vi "Save to binary file.vi"(6 "# saved frames out in":i32, 9 "Saving File":bool, 10 "Image array":u16[](array[numeric]), 11 "Byte Stream File in":refnum<file>) -> (2 "# saved frames out out":i32, 3 "Byte Stream File out":refnum<file>)   [LabVIEW 2011]
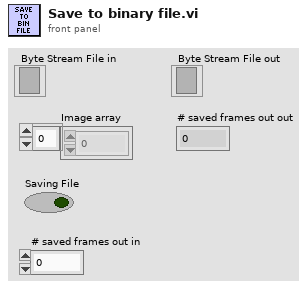
[diagram p1: front panel]
types:
  T1 = enum16{"big-endian, network order", "native, host order", "little-endian"}
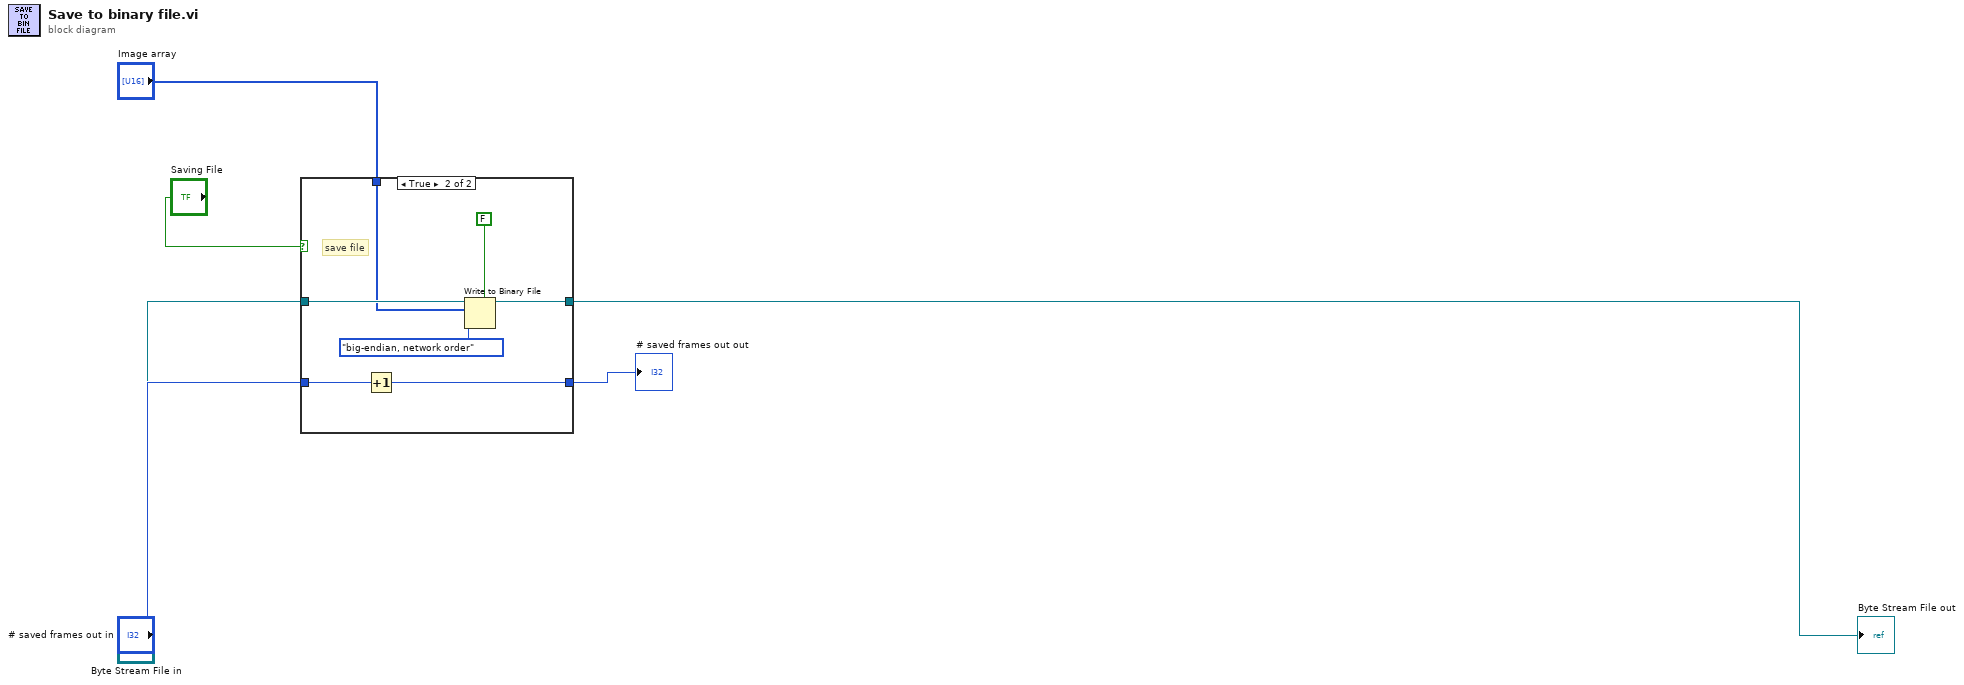
[diagram p0: block diagram]
diagram:
  n1 = case shown="True" "Saving File" {
    tunnel: [w8 w15] -> w1
    tunnel: "Byte Stream File in" -> [w8 w14]
    tunnel: "Image array" -> [_ w13]
    tunnel: "# saved frames out in" -> [w7 w10]
    tunnel: [w7 w9] -> w5
    frame False {
    }
    frame True {
      # "save file"
      n2 = Increment(x=w10) -> (x+1=w9:i32)
      n3 = Write to Binary File(file (use dialog)=w14, data=w13, 5:FALSE ("prepend array or string size? (T)"), 9:T1."big-endian, network order" ("byte order (0:big-endian, network order)")) -> (refnum out=w15:refnum<file>)  [unwired: 2 in, 2 out]
    }
  }
  "# saved frames out out" <- w5
  "Byte Stream File out" <- w1
